vi "Setpoint Decision Extension.vi"(11 "input cluster":T1) -> (3 "Setpoint":dbl)   [LabVIEW 2011]
uses:
  Robot Global Data.vi
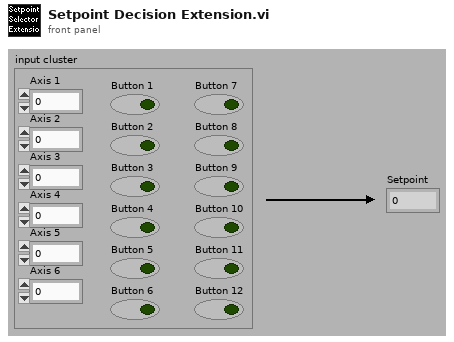
[diagram p1: front panel]
types:
  T1 = cluster{"Axis 1":dbl, "Axis 2":dbl, "Axis 3":dbl, "Axis 4":dbl, "Axis 5":dbl, "Axis 6":dbl, "Button 1":bool, "Button 2":bool, "Button 3":bool, "Button 4":bool, "Button 5":bool, "Button 6":bool, "Button 7":bool, "Button 8":bool, "Button 9":bool, "Button 10":bool, "Button 11":bool, "Button 12":bool}
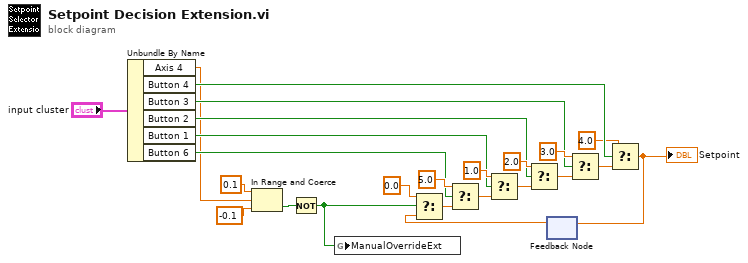
[diagram p0: block diagram]
diagram:
  n1 = Unbundle By Name("input cluster") -> ("Axis 4"=w9:dbl, "Button 4"=w14:bool, "Button 3"=w13:bool, "Button 2"=w15:bool, "Button 1"=w16:bool, "Button 6"=w11:bool)
  n2 = In Range and Coerce(upper limit=0.1, x=w9, lower limit=-0.1) -> (In Range?=w10:bool)  [unwired: 1 out]
  n3 = Not(x=w10) -> (.not. x?=w1:bool)
  n4 = global write "Robot Global Data.vi" "ManualOverrideExt"(w1) -> ()
  n5 = feedback #1() -> (w2:dbl)  [unwired: 1 out]
  n6 = Select(t=0.0, s=w1, f=w2) -> (s? t:f=w6:dbl)
  n7 = Select(t=5.0, s=w11, f=w6) -> (s? t:f=w17:dbl)
  n8 = Select(t=1.0, s=w16, f=w17) -> (s? t:f=w23:dbl)
  n9 = Select(t=2.0, s=w15, f=w23) -> (s? t:f=w22:dbl)
  n10 = Select(t=3.0, s=w13, f=w22) -> (s? t:f=w21:dbl)
  n11 = Select(t=4.0, s=w14, f=w21) -> (s? t:f=w3:dbl)
  "Setpoint" <- w3
  n12 = feedback-in #1(w3) -> ()
